vi "SetStateMask.vi"(8 "error in (no error)":errorcluster caption="Fehler (Eingang, kein Fehler)", 10 "mask":u16, 11 "device":u32) -> (0 "error out":errorcluster caption="Fehler (Ausgang)", 3 "function return":u32(ring))   [LabVIEW 2015, in "IRB.lvlib"]
doc: "irb_result IRB_EXPORT irb_set_state_mask(irb_device* device, uint16_t mask);"
uses:
  IRB.lvlib
  IRB.dll
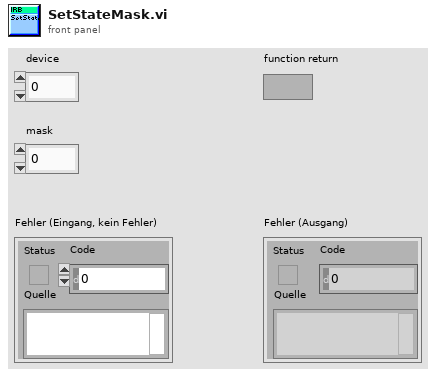
[diagram p1: front panel]
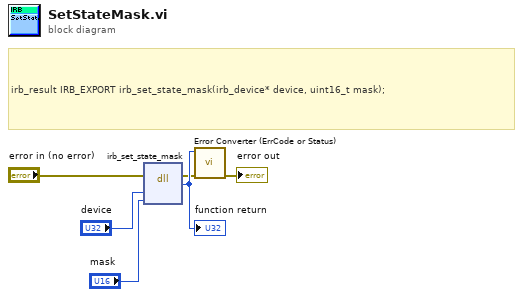
[diagram p0: block diagram]
diagram:
  # "irb_result IRB_EXPORT irb_set_state_mask(irb_device* device, uint16_t mask);"
  n1 = dll-call lib="C:/LabView/IRB/x86_32/IRB.*" fn="irb_set_state_mask"(error in="error in (no error)", "device"="device", "mask"="mask") -> (error out=w2:errorcluster, "return type"=w6:u32)  [unwired: 4 in, 1 out]
  "function return" <- w6
  n2 = call "Error Converter (ErrCode or Status).vi"("error in (no error)"=w2, "error code"=w6) -> ("error out"=→"error out":errorcluster)  [unwired: 9 in]
